vi "8-Bit Down Counter Controller.vi"(7 "Input":u8, 8 "Decrement":bool, 9 "Load":bool, 11 "Value":u8) -> (3 "Value+":u8)   [LabVIEW 2016]
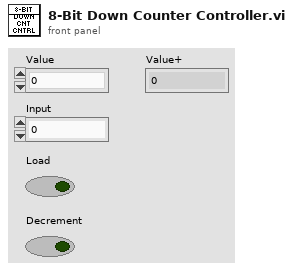
[diagram p1: front panel]
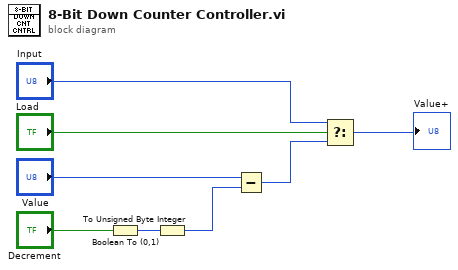
[diagram p0: block diagram]
diagram:
  n1 = Boolean To (0,1)(Boolean="Decrement") -> (0, 1=w4:i16)
  n2 = To Unsigned Byte Integer(number=w4) -> (unsigned 8bit integer=w3:u8)
  n3 = Subtract(x="Value", y=w3) -> (x-y=w2:u8)
  n4 = Select(t="Input", s="Load", f=w2) -> (s? t:f=→"Value+":u8)
